vi "Login.vi"() -> ()   [LabVIEW 2013]
uses:
  <vilib>/event_ctls.llb/eventvkey.ctl
panel:
  in  "Password":string
  in  "UserName":string
  in  "错误输入":errorcluster
  out "错误输出":errorcluster
  in  "Cancel":bool
  in  "OK":bool
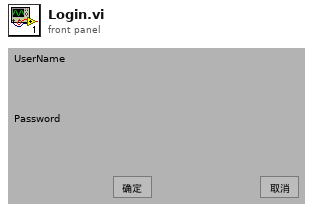
[diagram p1: front panel]
types:
  T1 = typedef "eventvkey.ctl" = enum16{"ASCII", "Enter", "Return", "Shift", "Ctrl", "Alt", "Cmd", "Opt", "Caps", "NumLock", "Clear", "Break", "Up", "Down", "Left", "Right", "Insert", "Delete", "Home", "End", "PageUp", "PageDown", "Escape", "Help", "Pause", "ScrollLock", "F1", "F2", "F3", "F4", "F5", "F6", "F7", "F8", "F9", "F10", "F11", "F12", "F13", "F14", "F15", "F16", "F17", "F18", "F19", "F20", "F21", "F22", "F23", "F24", "Play", "VolumeUp", "VolumeDown", "Mute", "Two Byte Char"}
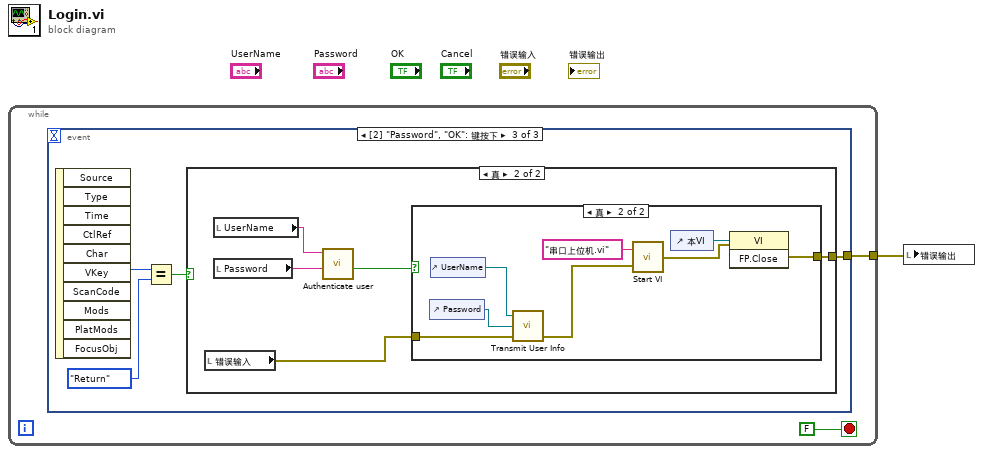
[diagram p0: block diagram]
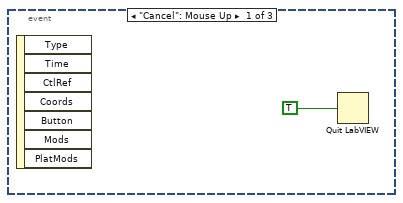
[diagram p2: hidden frame]
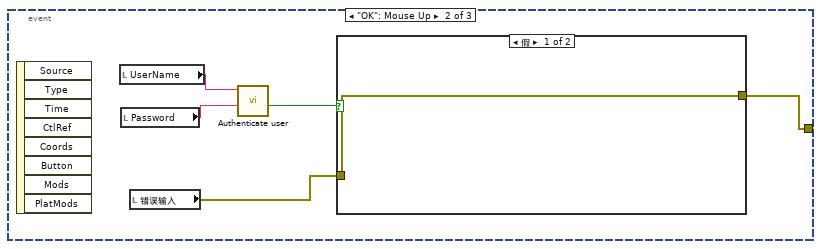
[diagram p3: hidden frame]
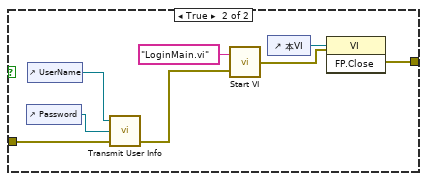
[diagram p4: hidden frame]
diagram:
  n1 = while {
    tunnel: [w2] -> w1
    stop <- FALSE stop-if-true
    n2 = event shown="[2] \"Password\", \"OK\": 键按下" {
      selector: _ -> [_ _ _]
      dyn-events: _ -> [_ _ _]
      timeout: _ -> [_ _ _]
      tunnel: [_ w9 w19] -> w2
      event "Cancel": Mouse Up {
        n3 = event-data() -> ()  [unwired: 1 in, 7 out]
        n4 = Quit LabVIEW(quit? (T)=TRUE ("退出？(T)")) -> ()
      }
      event "OK": Mouse Up {
        n5 = event-data() -> ()  [unwired: 1 in, 8 out]
        n6 = local read "UserName"() -> (w6:string)
        n7 = local read "Password"() -> (w5:string)
        n8 = local read "错误输入"() -> (w8:errorcluster)
        n9 = call "Authenticate user.vi"("Password"=w5, "Login"=w6) -> ("Verified?"=w7:bool)  [unwired: 5 in]
        n10 = case shown="假" w7 {
          tunnel: [w10 w12] -> w9
          tunnel: w8 -> [w10 w15]
          frame False {
          }
          frame True {
            n11 = control-ref of="Password"() -> (w13:refnum<vi>)
            n12 = control-ref of="UserName"() -> (w14:refnum<vi>)
            n13 = call "Transmit User Info.vi"("错误输入"=w15, "Password"=w13, "UserName"=w14) -> ("error out"=w11:errorcluster)  [unwired: 2 in]
            n14 = call "Start VI.vi"("错误输入（无错误）"=w11, "VI名称或相对路径"="LoginMain.vi" ("名称或相对路径")) -> ("error out"=w16:errorcluster)
            n15 = control-ref of="本VI"() -> (w17:refnum<vi>)
            n16 = invoke class="VI" method="FP.Close"(reference=w17, error in=w16) -> (error out=w12:errorcluster)  [unwired: 1 in, 2 out]
          }
        }
      }
      event "Password", "OK": Key Down {
        n17 = event-data() -> ("VKey"=w21:T1)  [unwired: 1 in, 9 out]
        n18 = Equal?(x=w21, y=eventvkey."Return") -> (x = y?=w22:bool)
        n19 = case shown="真" w22 {
          tunnel: [_ w26] -> w19
          frame False {
          }
          frame True {
            n20 = local read "错误输入"() -> (w27:errorcluster)
            n21 = local read "UserName"() -> (w24:string)
            n22 = local read "Password"() -> (w23:string)
            n23 = call "Authenticate user.vi"("Password"=w23, "Login"=w24) -> ("Verified?"=w25:bool)  [unwired: 5 in]
            n24 = case shown="真" w25 {
              tunnel: [w28 w30] -> w26
              tunnel: w27 -> [w28 w33]
              frame False {
              }
              frame True {
                n25 = control-ref of="Password"() -> (w31:refnum<vi>)
                n26 = control-ref of="UserName"() -> (w32:refnum<vi>)
                n27 = call "Transmit User Info.vi"("错误输入"=w33, "Password"=w31, "UserName"=w32) -> ("error out"=w29:errorcluster)  [unwired: 2 in]
                n28 = call "Start VI.vi"("错误输入（无错误）"=w29, "VI名称或相对路径"="串口上位机.vi" ("名称或相对路径")) -> ("error out"=w34:errorcluster)
                n29 = control-ref of="本VI"() -> (w35:refnum<vi>)
                n30 = invoke class="VI" method="FP.Close"(reference=w35, error in=w34) -> (error out=w30:errorcluster)  [unwired: 1 in, 2 out]
              }
            }
          }
        }
      }
    }
  }
  n31 = local write "错误输出"(w1) -> ()
